vi "ble_parse_heart_rate_measurement.vi"(8 "error in (no error)":errorcluster, 10 "Handle table":string[][](array[string]), 11 "payload":u8[](array[numeric])) -> (0 "error out":errorcluster, 2 "RR (ms)":dbl, 3 "HR (bpm)":u16)   [LabVIEW 2013]
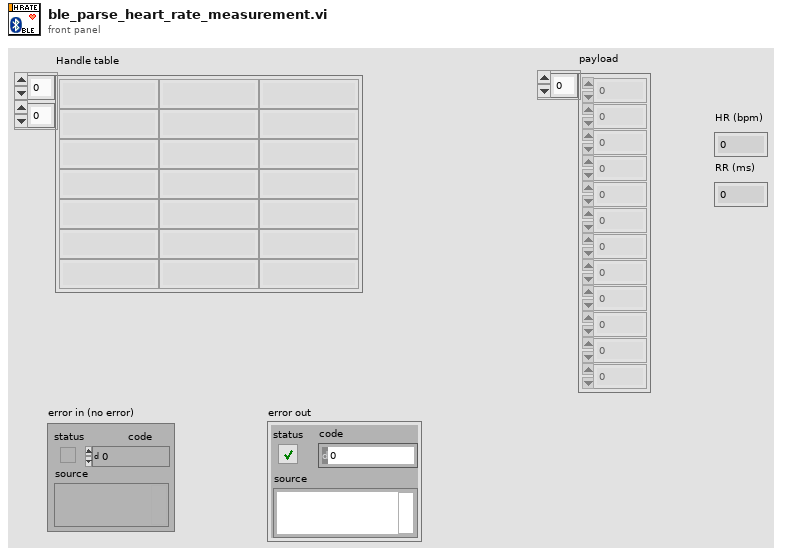
[diagram p1: front panel]
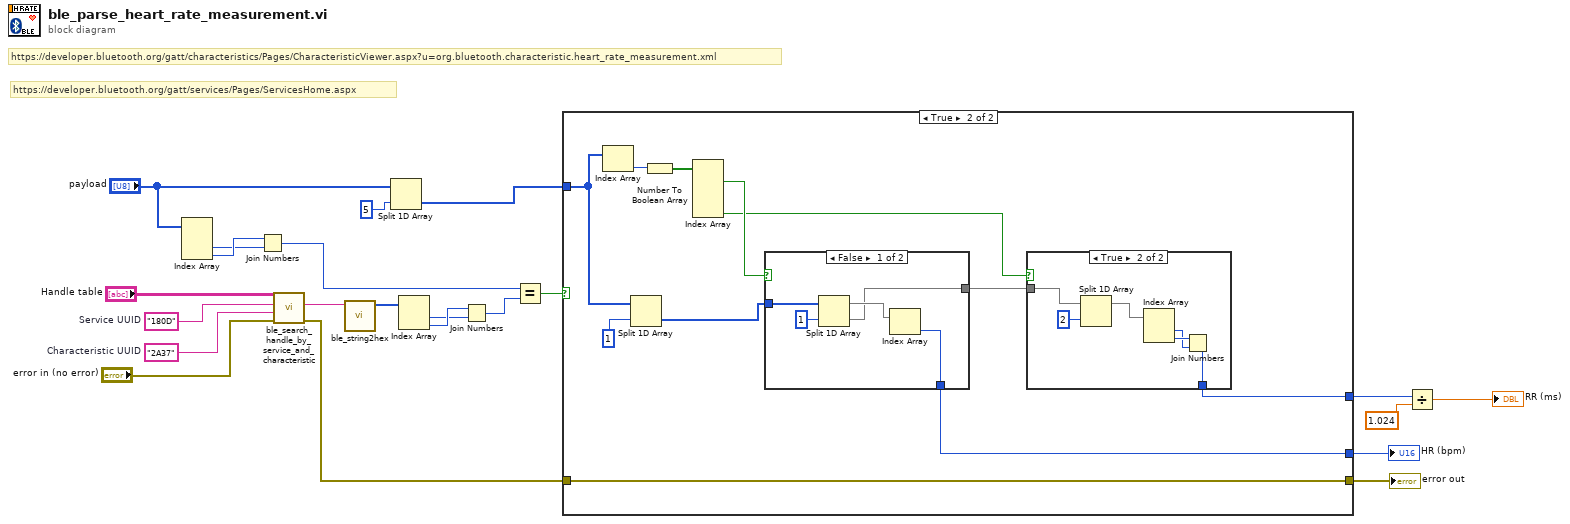
[diagram p0: block diagram]
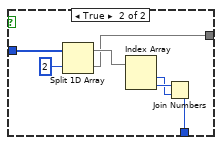
[diagram p4: hidden frame]
diagram:
  w20 = "2A37"  # Characteristic UUID
  w21 = "180D"  # Service UUID
  # "https://developer.bluetooth.org/gatt/services/Pages/ServicesHome.aspx"
  # "https://developer.bluetooth.org/gatt/characteristics/Pages/CharacteristicViewer.aspx?u=org.bluetooth.characteristic.heart_rate_measurement.xml"
  n1 = Index Array(array="payload") -> (element #2=w13:u8, element #3=w14:u8)  [unwired: 3 in, 1 out]
  n2 = Join Numbers(hi=w14, lo=w13) -> ((hi.lo)=w11:u16)
  n3 = call "ble_search_handle_by_service_and_characteristic.vi"("error in (no error)"="error in (no error)", "Characteristic UUID"=w20, "Service UUID"=w21, "Handle table"="Handle table") -> ("error out"=w9:errorcluster, "Handle"=w15:string)  [unwired: 6 in]
  n4 = call "ble_string2hex.vi"("HEX string IN"=w15) -> ("Byte Array IN (index0 LS byte)"=w18:u8[])  [unwired: 10 in]
  n5 = Split 1D Array(array="payload", index=5) -> (second subarray=w5:u8[])  [unwired: 1 out]
  n6 = Index Array(array=w18) -> (element #1=w16:u8, element #2=w17:u8)  [unwired: 2 in]
  n7 = Join Numbers(hi=w17, lo=w16) -> ((hi.lo)=w12:u16)
  n8 = Equal?(x=w11, y=w12) -> (x = y?=w10:bool)
  n9 = case shown="True" w10 {
    tunnel: w5 -> [_ w26]
    tunnel: w9 -> [w23 w34]
    tunnel: [w23 w34] -> w8
    tunnel: [_ w30] -> w4
    tunnel: [_ w27] -> w3
    frame False {
    }
    frame True {
      n10 = Index Array(array=w26) -> (element=w33:u8)  [unwired: 1 in]
      n11 = Split 1D Array(array=w26, index=1) -> (second subarray=w25:u8[])  [unwired: 1 out]
      n12 = Number To Boolean Array(number=w33) -> (Boolean array=w32:bool[])
      n13 = Index Array(array=w32) -> (element #1=w31:bool, element #5=w29:bool)  [unwired: 5 in, 3 out]
      n14 = case shown="False" w31 {
        tunnel: w25 -> [w43 w52]
        tunnel: [w42 w47] -> w30
        tunnel: [w41 w46] -> w28
        frame False {
          n15 = Split 1D Array(array=w43, index=1) -> (first subarray=w44:u8[], second subarray=w41:u8[])
          n16 = Index Array(array=w44) -> (element=w42:u8)  [unwired: 1 in]
        }
        frame True {
          n17 = Split 1D Array(array=w52, index=2) -> (first subarray=w50:u8[], second subarray=w46:u8[])
          n18 = Index Array(array=w50) -> (element #1=w48:u8, element #2=w49:u8)  [unwired: 2 in]
          n19 = Join Numbers(hi=w49, lo=w48) -> ((hi.lo)=w47:u16)
        }
      }
      n20 = case shown="True" w29 {
        tunnel: w28 -> [_ w40]
        tunnel: [_ w35] -> w27
        frame False {
        }
        frame True {
          n21 = Split 1D Array(array=w40, index=2) -> (first subarray=w38:u8[])  [unwired: 1 out]
          n22 = Index Array(array=w38) -> (element #1=w36:u8, element #2=w37:u8)  [unwired: 2 in]
          n23 = Join Numbers(hi=w37, lo=w36) -> ((hi.lo)=w35:u16)
        }
      }
    }
  }
  "error out" <- w8
  "HR (bpm)" <- w4
  n24 = Divide(x=w3, y=1.024) -> (x/y=→"RR (ms)":dbl)
